vi "Get Number of RUNs.vi"(8 "error in (no error)":errorcluster, 11 "Schedule Block in":refnum<class "Schedule Block.lvclass">) -> (0 "error out":errorcluster, 2 "No. of RUNs":i32, 3 "Schedule Block out":refnum<class "Schedule Block.lvclass">)   [LabVIEW 2020, in "TALOS.lvlib" / "Run Utilities.lvlib" / "Schedule Block.lvclass"]
uses:
  Schedule Block.lvclass
  Schedule Block.lvclass/Schedule Block.ctl
  Schedule/Schedule.lvclass
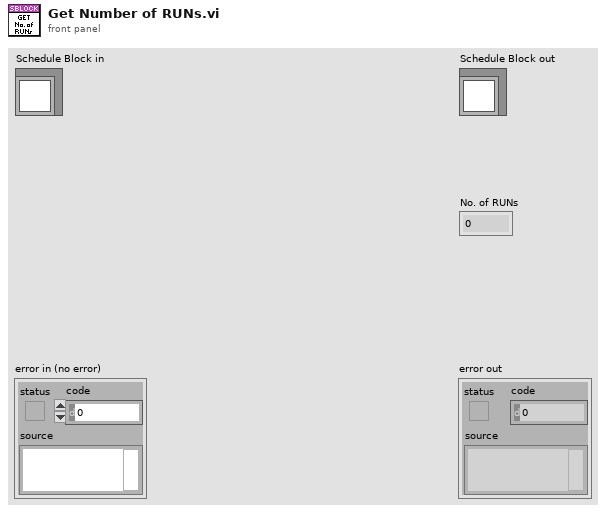
[diagram p1: front panel]
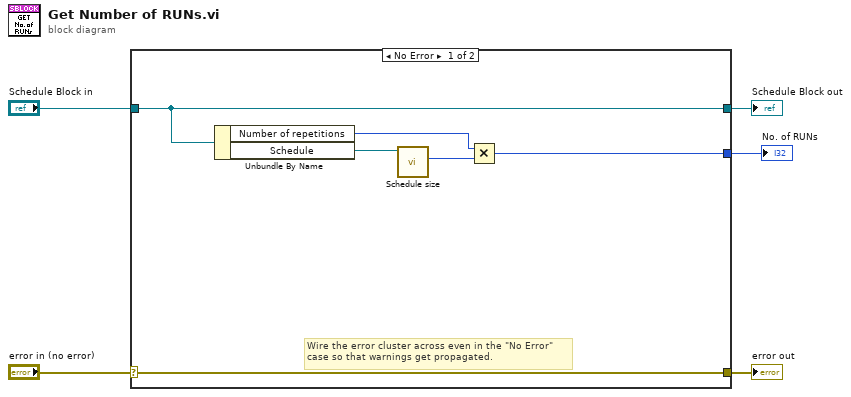
[diagram p0: block diagram]
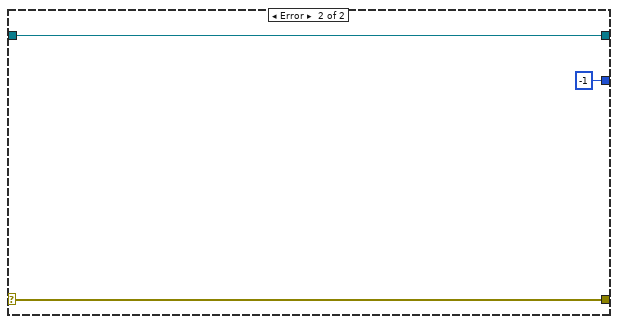
[diagram p2: hidden frame]
diagram:
  n1 = case shown="No Error" "error in (no error)" {
    selector: "error in (no error)" -> [w11 w14]
    tunnel: [w11 w14] -> w4
    tunnel: [w10 w13] -> w2
    tunnel: "Schedule Block in" -> [w10 w13]
    tunnel: [w6 -1] -> w1
    frame No Error {
      # "Wire the error cluster across even in the \"No Error\"\ncase so that warnings get propagated."
      n2 = Unbundle By Name(w10) -> ("Number of repetitions"=w8:u16, "Schedule"=w9:refnum<class "Schedule.lvclass">)
      n3 = call-dynamic "Schedule size.vi"("Schedule in"=w9) -> ("Size"=w7:i32)  [unwired: 8 in, 2 out]
      n4 = Multiply(x=w8, y=w7) -> (x*y=w6:i32)
    }
    frame Error {
    }
  }
  "error out" <- w4
  "Schedule Block out" <- w2
  "No. of RUNs" <- w1
